vi "initialize timing source.vi"(8 "error in":errorcluster, 11 "timing source in":refnum<class "absolute usec timing source.lvclass">) -> (0 "error out":errorcluster, 3 "timing source out":refnum<class "absolute usec timing source.lvclass">)   [LabVIEW 2013, in "absolute usec timing source.lvclass"]
doc: "An interface for initializing a timing source. In many cases this may be a no-op. There is no expectation about when this function should be called, but it must be called before entering the loop to be timed."
uses:
  absolute usec timing source.lvclass
  absolute usec timing source.lvclass/absolute usec timing source.ctl
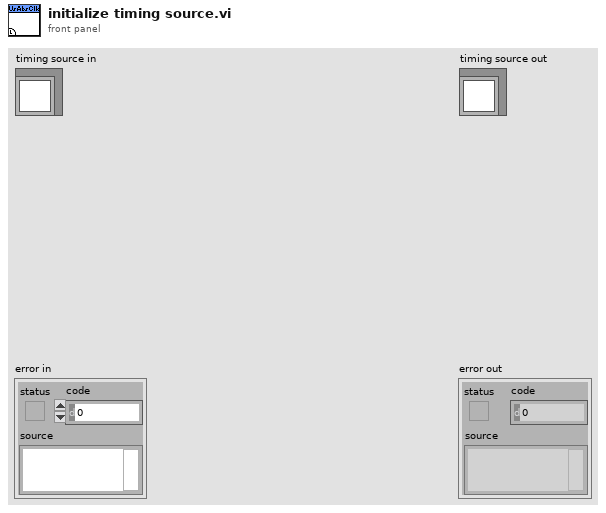
[diagram p1: front panel]
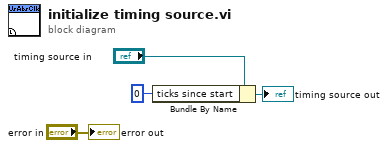
[diagram p0: block diagram]
diagram:
  n1 = Bundle By Name(cluster="timing source in", "ticks since start"=i64 0) -> (→"timing source out":refnum<class "absolute usec timing source.lvclass">)
  "error out" <- "error in"
